vi "例3.5 利用“匹配正则表达式”进行字符串的分解.vi"() -> ()   [LabVIEW 2012]
uses:
  <vilib>/regexp/Match Regular Expression.xnode
panel:
  out "数字":dbl
  out "匹配之后":string
  out "所有匹配":string
  out "匹配之前":string
  in  "输入字符串":string="VOLTS DC +1.345E+02"
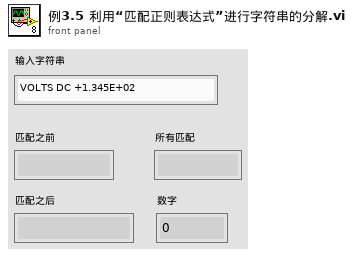
[diagram p1: front panel]
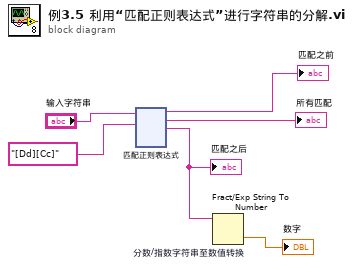
[diagram p0: block diagram]
diagram:
  n1 = xnode "匹配正则表达式"("输入字符串"="输入字符串", "正则表达式"="[Dd][Cc]") -> ("匹配之前"=→"匹配之前":string, "所有匹配"=→"所有匹配":string, "匹配之后"=w3:string)  [unwired: 4 in, 2 out]
  "匹配之后" <- w3
  n2 = Fract/Exp String To Number "分数/指数字符串至数值转换"(string=w3) -> (number=→"数字":dbl)  [unwired: 3 in, 1 out]
